vi "Update.vi"(8 "Diffuse Colour":u32(colorbox), 9 "Object Index":i32, 10 "Pixel Data in":u32[][](array[numeric]), 11 "Scene in":refnum<class "Scene.lvclass">) -> (2 "Pixel Data out":u32[][](array[numeric]), 3 "Scene out":refnum<class "Scene.lvclass">)   [LabVIEW 2022 SP3, in "Application.lvlib" / "Scene.lvclass"]
uses:
  Scene.lvclass
  Scene.lvclass/Scene.ctl
  Transform And Project.vi/196e4586-e654-41ec-a3a4-43fea5068e8e.vi
  Transform And Project.vi/a59a4b44-279f-4314-be75-e28f6a03f0ec.vi
  Libraries/3D/Normal.vi
  Libraries/3D/Project And Illuminate Triangle.vi
  Libraries/3D/Apply View Matrix.vi
  Libraries/3D/Transform Triangle.vi
  Libraries/3D/Sort Triangles.vi
  Raster.vi/edb3f0c2-b950-4a44-8897-096d76b30880.vi
  Raster.vi/76d78098-f527-454b-a08a-aac5a717328f.vi
  <vilib>/Utility/High Resolution Relative Seconds.vi
  Libraries/3D/Normalise Vector.vi
  Libraries/3D/Multiply Vector By Matrix.vi
  Libraries/3D/Scale Point 3D (SGL) To Screen.vi
  Libraries/3D/Calculate Triangle Illumination.vi
  Libraries/3D/Calculate View Matrix.vi
  Sub Vs/Create Translation Matrix.vi
  Sub Vs/Create Z Rotation Matrix.vi
  Sub Vs/Create Y Rotation Matrix.vi
  Sub Vs/Create X Rotation Matrix.vi
  <vilib>/Utility/colorconv.llb/Color to RGB.vi
  Libraries/3D/Dot Product.vi
  <vilib>/Utility/colorconv.llb/RGB to Color.vi
  <userlib>/_OpenG.lib/array/array.llb/Sort Array__ogtk.vi
  <userlib>/_OpenG.lib/array/array.llb/Sort 1D Array (SGL)__ogtk.vi
  Libraries/Utility/Utility.lvlib
  <vilib>/ptbypt/NI_PtbyPt.lvlib
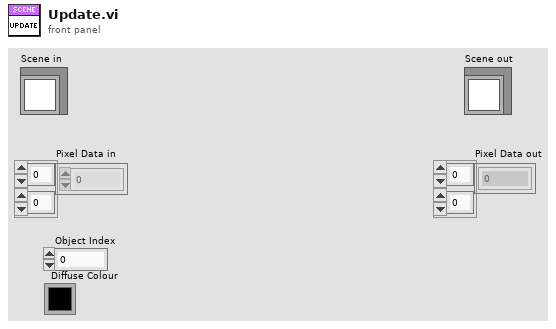
[diagram p1: front panel]
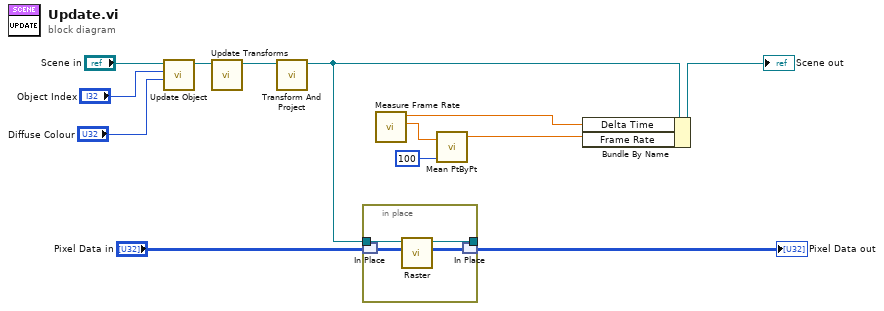
[diagram p0: block diagram]
diagram:
  n1 = call "Update Object.vi"("Diffuse Colour"="Diffuse Colour", "Object Index"="Object Index", "Scene in"="Scene in") -> ("Scene out"=w3:refnum<class "Scene.lvclass">)  [unwired: 8 in]
  n2 = call "Update Transforms.vi"("Scene in"=w3) -> ("Scene out"=w5:refnum<class "Scene.lvclass">)  [unwired: 10 in]
  n3 = call "Transform And Project.vi"("Scene in"=w5) -> ("Scene out"=w9:refnum<class "Scene.lvclass">)  [unwired: 10 in]
  n4 = in-place {
    in-place-border: w9 -> [w15]
    in-place-border: [w14] -> _
    n5 = in-place-match #1("Pixel Data in") -> (w17:u32[][])
    n6 = call "Raster.vi"("Pixel Data in"=w17, "Scene in"=w15) -> ("Pixel Data out"=w16:u32[][], "Scene out"=w14:refnum<class "Scene.lvclass">)  [unwired: 8 in]
    n7 = in-place-match #1(w16) -> (→"Pixel Data out":u32[][])
  }
  n8 = call "Measure Frame Rate.vi"() -> ("Frame Rate [FPS]"=w11:dbl, "Delta Time [s]"=w6:dbl)  [unwired: 10 in]
  n9 = call <vilib>:"Mean PtByPt.vi"("x"=w11, "sample length"=100) -> ("mean"=w7:dbl)  [unwired: 2 in, 1 out]
  n10 = Bundle By Name(cluster=w9, "Delta Time"=w6, "Frame Rate"=w7) -> (→"Scene out":refnum<class "Scene.lvclass">)
